vi "FT_Get_Device_Info_Detail.vi"(0 "Device Index":u32) -> (1 "FT_Status":u32(ring) items=["FT_OK", "FT_INVALID_HANDLE", "FT_DEVICE_NOT_FOUND", "FT_DEVICE_NOT_OPENED", "FT_IO_ERROR", "FT_INSUFFICIENT_RESOURCES", "FT_INVALID_PARAMETER", "FT_INVALID_BAUD_RATE", "FT_DEVICE_NOT_OPENED_FOR_ERASE", "FT_DEVICE_NOT_OPENED_FOR_WRITE", "FT_FAILED_TO_WRITE_DEVICE", "FT_EEPROM_READ_FAILED", "FT_EEPROM_WRITE_FAILED", "FT_EEPROM_ERASE_FAILED", "FT_EEPROM_NOT_PRESENT", "FT_EEPROM_NOT_PROGRAMMED", "FT_INVALID_ARGS", "FT_NOT_SUPPORTED", "FT_OTHER_ERROR"], 2 "Device Info Node":T1 {"FT_Handle" format="%.0x"; "LocID" format="%.0x"; "PID" format="%.0x"; "VID" format="%.0x"; "Type" items=["FT232B-FT245B", "FT8U232AM-FT8U245AM", "FT8U100AX", "UNKNOWN", "FT2232", "FT232R", "FT2232H", "FT4232H", "FT232H"]})   [LabVIEW 2019]
uses:
  FTD2XX.dll
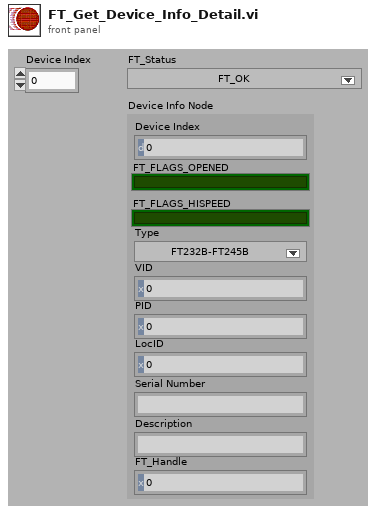
[diagram p1: front panel]
types:
  T1 = cluster{"Device Index":u32, "FT_FLAGS_OPENED":bool, "FT_FLAGS_HISPEED":bool, "Type":u32, "VID":u32, "PID":u32, "LocID":i32, "Serial Number":string, "Description":string, "FT_Handle":u32}
  T2 = cluster{"Device Index":u32, bool, bool, "Type":u32, u32, u32, "LocID":i32, "Serial Number":string, "Description":string, "FT_Handle":u32}
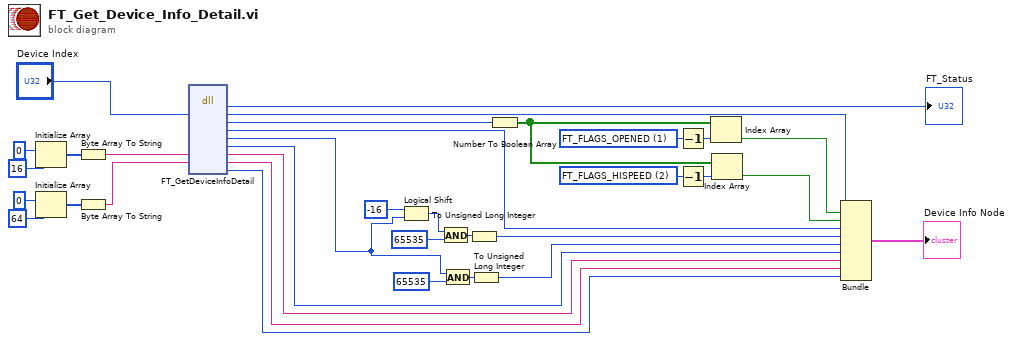
[diagram p0: block diagram]
diagram:
  w1 = u32 2 items=["FT_FLAGS_OPENED"=1, "FT_FLAGS_HISPEED"=2] ("Flags")
  w4 = u32 1 items=["FT_FLAGS_OPENED"=1, "FT_FLAGS_HISPEED"=2] ("Flags")
  n1 = Initialize Array(u8 0, 16 ("dimension size")) -> (w27:u8[])
  n2 = Initialize Array(u8 0, 64 ("dimension size")) -> (w25:u8[])
  n3 = Byte Array To String(unsigned byte array=w27) -> (string=w24:string)
  n4 = Byte Array To String(unsigned byte array=w25) -> (string=w23:string)
  n5 = dll-call lib="FTD2XX.dll" fn="FT_GetDeviceInfoDetail"("Device Index"="Device Index", "Serial Number"=w24, "Description"=w23) -> ("FT_Status"=→"FT_Status":u32, "Device Index"=w32:u32, "Flags"=w9:u32, "Type"=w31:u32, "Device ID"=w10:u32, "LocID"=w11:i32, "Serial Number"=w30:string, "Description"=w12:string, "FT_Handle"=w29:u32)  [unwired: 8 in, 2 out]
  n6 = Logical Shift(y=-16, x=w10) -> (x << y=w18:u32)
  n7 = And(x=w18, y=u32 65535) -> (x .and. y?=w16:u32)
  n8 = And(x=w10, y=u32 65535) -> (x .and. y?=w14:u32)
  n9 = To Unsigned Long Integer(number=w16) -> (unsigned 32bit integer=w15:u32)
  n10 = To Unsigned Long Integer(number=w14) -> (unsigned 32bit integer=w13:u32)
  n11 = Number To Boolean Array(number=w9) -> (Boolean array=w7:bool[])
  n12 = Decrement(x=w4) -> (x-1=w3:u32)
  n13 = Decrement(x=w1) -> (x-1=w2:u32)
  n14 = Index Array(array=w7, index=w3) -> (element=w8:bool)
  n15 = Index Array(array=w7, index=w2) -> (element=w6:bool)
  n16 = Bundle("Device Index"=w32, w8, w6, "Type"=w31, w15, w13, "LocID"=w11, "Serial Number"=w30, "Description"=w12, "FT_Handle"=w29) -> (→"Device Info Node":T2)  [unwired: 1 in]
